vi "RDV-GUI-SinglePlot.vi"() -> ()   [LabVIEW 2020, in "RDV-Reflection_Data_viewer.lvclass"]
uses:
  RDV-Reflection_Data_viewer.lvclass
  RDV-PRELAUNCH_DATA.ctl
  RDV-XY_GRAPH_REFS.ctl
  RDV-GUI_REFS.ctl
panel:
  in  "Autoscale":bool
  in  "refl Imag":bool
  in  "refl Real":bool
  in  "Perm Imag":bool
  in  "Perm Real":bool
  in  "Toggle Plot":bool
  in  "Stop":bool
  out "error out":errorcluster
  in  "Folder Path":path=path "C:/projects/Universitet/Master/data/Real Test - First libreVNA test with calibration file/Converted Data"
  out "Data":T1(graph)
  # "Reflection"
  # "Permativity"
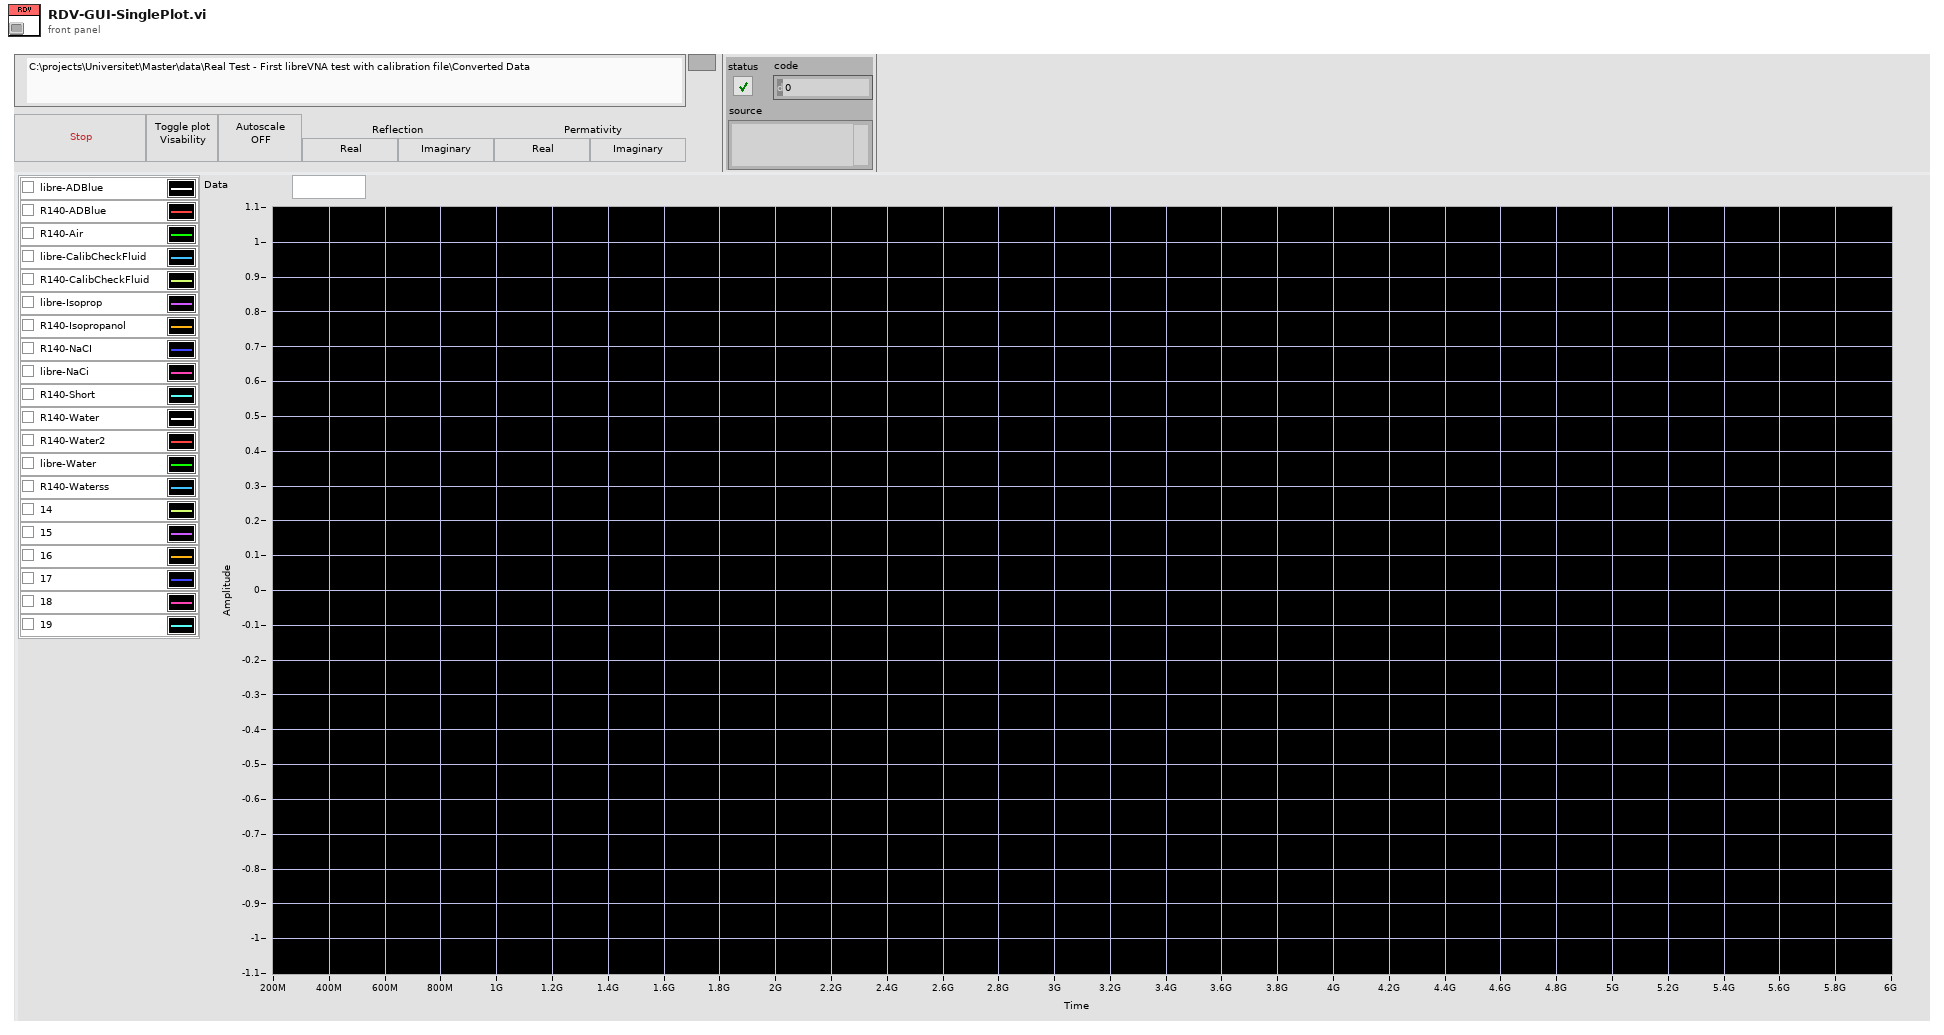
[diagram p1: front panel]
types:
  T1 = cluster{"Frequency":dbl[], "Reflection'":dbl[]}[]
  T2 = typedef "RDV-Reflection_Data_viewer.lvclass/RDV-PRELAUNCH_DATA.ctl" = cluster{"XY graph refs":T3, "GUI Refs":T4}
  T3 = typedef "RDV-Reflection_Data_viewer.lvclass/RDV-XY_GRAPH_REFS.ctl" = cluster{"Reflection Real":refnum<vi>, "Reflection Imag":refnum<vi>, "Permittivity Real":refnum<vi>, "Permittivity Imag":refnum<vi>}
  T4 = typedef "RDV-Reflection_Data_viewer.lvclass/RDV-GUI_REFS.ctl" = cluster{"Autoscale":refnum<vi>, "plot Selector":refnum<vi>[]}
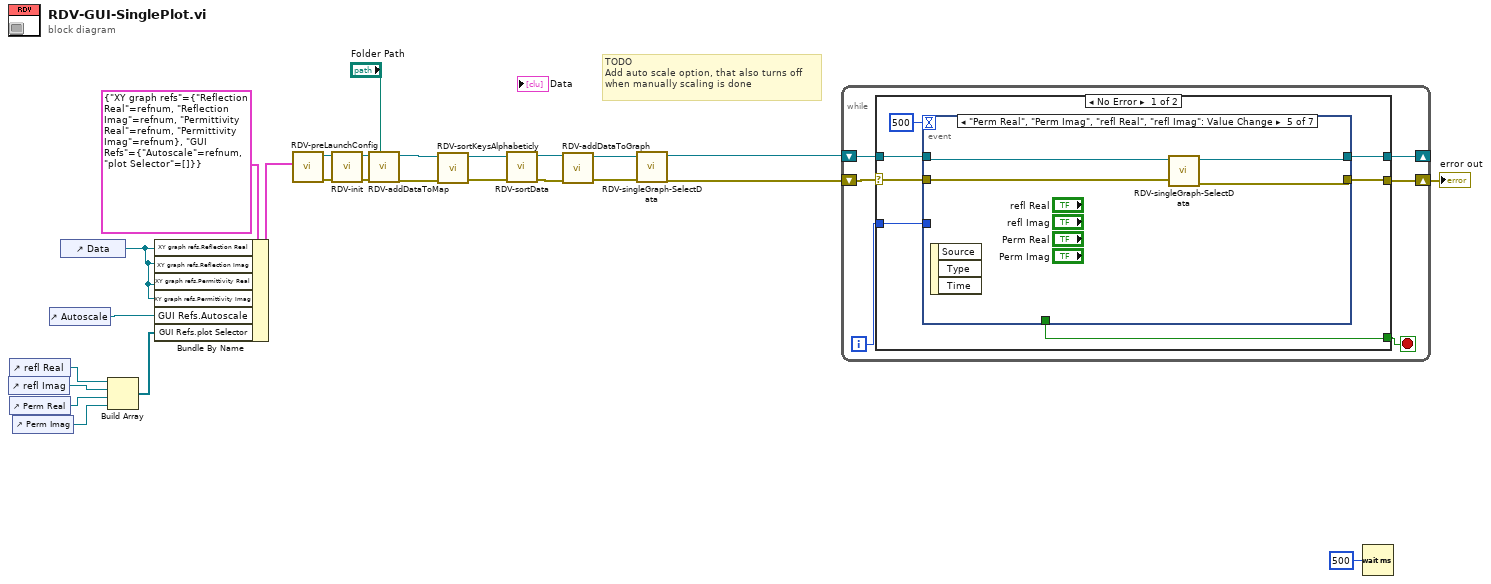
[diagram p0: block diagram]
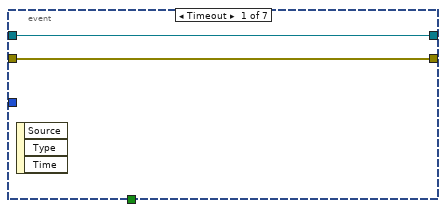
[diagram p2: hidden frame]
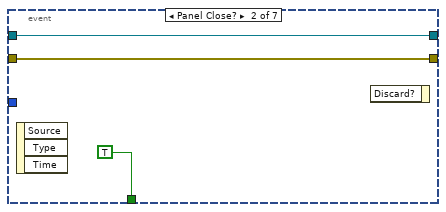
[diagram p3: hidden frame]
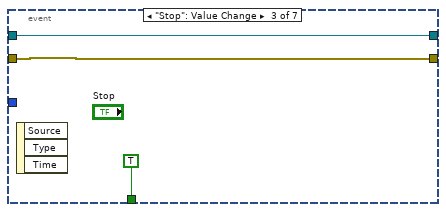
[diagram p4: hidden frame]
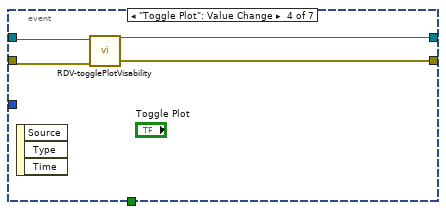
[diagram p5: hidden frame]
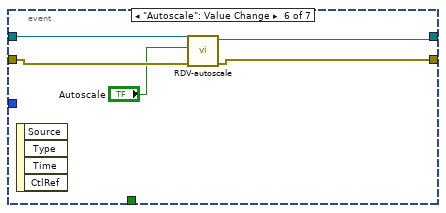
[diagram p6: hidden frame]
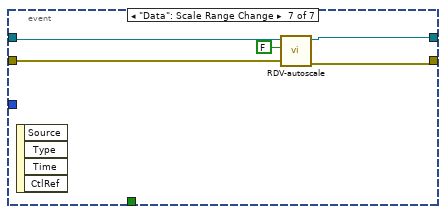
[diagram p7: hidden frame]
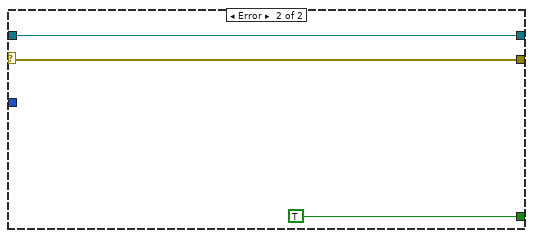
[diagram p8: hidden frame]
diagram:
  # "TODO\nAdd auto scale option, that also turns off\nwhen manually scaling is done"
  n1 = control-ref of="refl Imag"() -> (w3:refnum<vi>)
  n2 = control-ref of="refl Real"() -> (w4:refnum<vi>)
  n3 = control-ref of="Perm Real"() -> (w2:refnum<vi>)
  n4 = control-ref of="Perm Imag"() -> (w1:refnum<vi>)
  n5 = control-ref of="Autoscale"() -> (w6:refnum<vi>)
  n6 = control-ref of="Data"() -> (w11:refnum<vi>)
  n7 = Build Array(w4, w3, w2, w1) -> (w5:refnum<vi>[])
  n8 = Bundle By Name(cluster=T2 {"XY graph refs"={"Reflection Real"=refnum, "Reflection Imag"=refnum, "Permittivity Real"=refnum, "Permittivity Imag"=refnum}, "GUI Refs"={"Autoscale"=refnum, "plot Selector"=[]}} ("preLaunch Config"), "XY graph refs.Reflection Real"=w11, "XY graph refs.Reflection Imag"=w11, "XY graph refs.Permittivity Real"=w11, "XY graph refs.Permittivity Imag"=w11, "GUI Refs.Autoscale"=w6, "GUI Refs.plot Selector"=w5) -> (w17:T2)
  n9 = call "RDV-preLaunchConfig.vi"("preLaunch Config"=w17) -> ("error out"=w13:errorcluster, "RDV-Reflection_Data_viewer out"=w14:refnum<class "RDV-Reflection_Data_viewer.lvclass">)  [unwired: 9 in]
  n10 = call "RDV-init.vi"("error in (no error)"=w13, "RDV-Reflection_Data_viewer in"=w14) -> ("error out"=w15:errorcluster, "RDV-Reflection_Data_viewer out"=w16:refnum<class "RDV-Reflection_Data_viewer.lvclass">)  [unwired: 8 in]
  n11 = call "RDV-addDataToMap.vi"("Folder Path"="Folder Path", "error in (no error)"=w15, "RDV-Reflection_Data_viewer in"=w16) -> ("error out"=w19:errorcluster, "RDV-Reflection_Data_viewer out"=w25:refnum<class "RDV-Reflection_Data_viewer.lvclass">)  [unwired: 7 in]
  n12 = call "RDV-sortKeysAlphabeticly.vi"("error in (no error)"=w19, "RDV-Reflection_Data_viewer in"=w25) -> ("error out"=w20:errorcluster, "RDV-Reflection_Data_viewer out"=w24:refnum<class "RDV-Reflection_Data_viewer.lvclass">)  [unwired: 8 in]
  n13 = call "RDV-sortData.vi"("error in (no error)"=w20, "RDV-Reflection_Data_viewer in"=w24) -> ("error out"=w21:errorcluster, "RDV-Reflection_Data_viewer out"=w22:refnum<class "RDV-Reflection_Data_viewer.lvclass">)  [unwired: 8 in]
  n14 = call "RDV-addDataToGraph.vi"("error in (no error)"=w21, "RDV-Reflection_Data_viewer in"=w22) -> ("error out"=w7:errorcluster, "RDV-Reflection_Data_viewer out"=w10:refnum<class "RDV-Reflection_Data_viewer.lvclass">)  [unwired: 8 in]
  n15 = call "RDV-singleGraph-SelectData.vi"("error in (no error)"=w7, "RDV-Reflection_Data_viewer in"=w10) -> ("error out"=w8:errorcluster, "RDV-Reflection_Data_viewer out"=w9:refnum<class "RDV-Reflection_Data_viewer.lvclass">)  [unwired: 8 in]
  n16 = while {
    shift-right: [w31] -> _
    shift-left: w9 -> [w32]
    shift-right: [w29] -> w18
    shift-left: w8 -> [w30]
    i -> [w27]
    stop <- w28 stop-if-true
    n17 = case shown="No Error" w30 {
      selector: w30 -> [w36 w67]
      tunnel: w32 -> [w37 w68]
      tunnel: [w39 w68] -> w31
      tunnel: [w38 w67] -> w29
      tunnel: [w34 TRUE ("stop")] -> w28
      tunnel: w27 -> [w33 _]
      frame No Error {
        n18 = event shown="[4] \"Perm Real\", \"Perm Imag\", \"refl Real\", \"refl Imag\": Value Change" {
          selector: _ -> [_ _ _ _ _ _ _]
          dyn-events: _ -> [_ _ _ _ _ _ _]
          timeout: 500 -> [_ _ _ _ _ _ _]
          tunnel: [w41 w43 w46 w51 w55 w57 w65] -> w39
          tunnel: w37 -> [w41 w43 w46 w48 w54 w59 w64]
          tunnel: [w40 w42 w45 w50 w52 w58 w62] -> w38
          tunnel: w36 -> [w40 w42 w45 w49 w53 w60 w63]
          tunnel: [_ TRUE ("Discard?") TRUE ("Discard?") _ _ _ _] -> w34
          tunnel: w33 -> [_ _ _ _ _ _ _]
          event Timeout {
            n19 = event-data() -> ()  [unwired: 1 in, 3 out]
          }
          event Panel Close? {
            n20 = event-data() -> ()  [unwired: 1 in, 3 out]
            n21 = event-data() -> ()  [unwired: 2 in, 1 out]
          }
          event "Stop": Value Change {
            n22 = event-data() -> ()  [unwired: 1 in, 3 out]
          }
          event "Toggle Plot": Value Change {
            n23 = event-data() -> ()  [unwired: 1 in, 3 out]
            n24 = call "RDV-togglePlotVisability.vi"("error in (no error)"=w49, "RDV-Reflection_Data_viewer in"=w48) -> ("error out"=w50:errorcluster, "RDV-Reflection_Data_viewer out"=w51:refnum<class "RDV-Reflection_Data_viewer.lvclass">)  [unwired: 8 in]
          }
          event "Perm Real", "Perm Imag", "refl Real", "refl Imag": Value Change {
            n25 = event-data() -> ()  [unwired: 1 in, 3 out]
            n26 = call "RDV-singleGraph-SelectData.vi"("error in (no error)"=w53, "RDV-Reflection_Data_viewer in"=w54) -> ("error out"=w52:errorcluster, "RDV-Reflection_Data_viewer out"=w55:refnum<class "RDV-Reflection_Data_viewer.lvclass">)  [unwired: 8 in]
          }
          event "Autoscale": Value Change {
            n27 = event-data() -> ()  [unwired: 1 in, 4 out]
            n28 = call "RDV-autoscale.vi"("error in (no error)"=w60, "Autoscale"="Autoscale", "RDV-Reflection_Data_viewer in"=w59) -> ("error out"=w58:errorcluster, "RDV-Reflection_Data_viewer out"=w57:refnum<class "RDV-Reflection_Data_viewer.lvclass">)  [unwired: 7 in]
          }
          event "Data": Scale Range Change {
            n29 = event-data() -> ()  [unwired: 1 in, 4 out]
            n30 = call "RDV-autoscale.vi"("error in (no error)"=w63, "Autoscale"=FALSE, "RDV-Reflection_Data_viewer in"=w64) -> ("error out"=w62:errorcluster, "RDV-Reflection_Data_viewer out"=w65:refnum<class "RDV-Reflection_Data_viewer.lvclass">)  [unwired: 7 in]
          }
        }
      }
      frame Error {
      }
    }
  }
  "error out" <- w18
  n31 = Wait (ms)(milliseconds to wait=u32 500) -> ()  [unwired: 1 out]
